vi "pulse.vi"(1 "i":i16, 2 "Start i":i16, 3 "Size":i16) -> (0 "Out":u16)   [LabVIEW 2010, in "Wall Follower.lvrbt"]
uses:
  Wall Follower.lvrbt
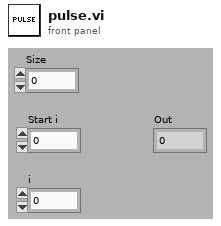
[diagram p1: front panel]
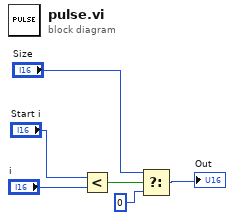
[diagram p0: block diagram]
diagram:
  n1 = Less?(x="Start i", y="i") -> (x < y?=w4:bool)
  n2 = Select(t="Size", s=w4, f=i16 0) -> (s? t:f=→"Out":i16)
